vi "JoyStick2.vi"() -> ()   [LabVIEW 2016]
panel:
  in  "JoyStick":bool
  out "X 2":bool
  out "Y 2":bool
  out "Z 2":bool
  out "LowSpeed?":bool
  out "down":string
  out "right":string
  out "Up":string
  out "left":string
  out "Boolean":bool
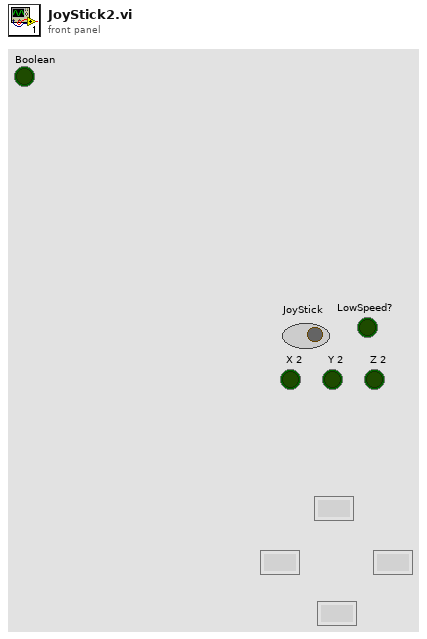
[diagram p1: front panel]
types:
  T1 = typedef "ControllerDiagPacket.ctl" = cluster{"Number of Diag Packets":i32, "Axes":T2[], "error":errorcluster}
  T2 = typedef "AxisDiagPacket.ctl" = cluster{"Axis Name":string, "Analog Input 0":dbl, "Analog Input 1":dbl, "Axis Fault (num)":i32, "Axis Fault (str)":string, "Axis Fault (bits)":cluster{"AmplifierFault":bool, "AmplifierTemperatureFault":bool, "CcwEndOfTravelLimitFault":bool, "CcwSoftwareLimitFault":bool, "CommunicationLostFault":bool, "CwEndOfTravelLimitFault":bool, "CwSoftwareLimitFault":bool, "EmergencyStopFault":bool, "EncoderFault":bool, "ExternalFault":bool, "FeedbackScalingFault":bool, "GantryMisalignFault ":bool, "HallSensorFault":bool, "InPositionTimeoutFault":bool, "InternalFault":bool, "MarkerSearchFault":bool, "MaxVelocityCommandFault":bool, "MissedInterruptFault":bool, "MotorTemperatureFault":bool, "None":bool, "OverCurrentFault":bool, "PositionErrorFault":bool, "PositionFeedbackFault":bool, "PowerSupplyFault":bool, "ProbeInputFault":bool, "SafeZoneFault":bool, "VelocityErrorFault":bool, "VelocityFeedbackFault":bool, "VoltageClampFault":bool}, "Axis Status (num)":i32, "Axis Status (str)":string, "Axis Status (bits)":cluster{"BacklashActive":bool, "CalibrationEnabled1D":bool, "CalibrationEnabled2D":bool, "CommandValid":bool, "DriveAbortPending":bool, "DrivePending":bool, "Enabling":bool, "GainMappingEnabled":bool, "GantryAligned":bool, "GantryRealigning":bool, "Homed":bool, "Homing":bool, "IFOVEnabled":bool, "JogGenerating":bool, "Jogging":bool, "JoystickControl":bool, "MasterSlaveControl":bool, "MotionBlocked":bool, "MotionClamped":bool, "MoveDone":bool, "None":bool, "NotVirtual":bool, "Profiling":bool, "Stability0":bool, "Stability1":bool, "TrajectoryFiltering":bool, "WaitDone":bool}, "Current Command":sgl, "Current Error":sgl, "Current Feedback":sgl, "Digital Inputs":i32, "Digital Outputs":i32, "Drive Status":i32, "Drive Status (str)":string, "Drive Status (bits)":cluster{"AccelerationPhase":bool, "AutofocusActive":bool, "BrakeOutput":bool, "CcwEndOfTravelLimitInput":bool, "CosineEncoderError":bool, "CurrentClamp":bool, "CwEndOfTravelLimitInput":bool, "DecelerationPhase":bool, "DualLoopActive":bool, "EmergencyStopInput":bool, "Enabled":bool, "EncoderClipping":bool, "GalvoCalibrationEnabled":bool, "GalvoPowerCorrection":bool, "HallAInput":bool, "HallBInput":bool, "HallCInput":bool, "HighResolutionMode":bool, "HomeLimitInput":bool, "InPosition":bool, "InPosition2":bool, "MarkerInput":bool, "MarkerLatch":bool, "MoveActive":bool, "NoMotorSupply":bool, "None":bool, "PowerLimiting":bool, "ProgrammingFlash":bool, "ProgrammingMXH":bool, "PSOHaltLatch":bool, "ServoControl":bool, "SineEncoderError":bool}, "Position Feedback Auxiliary":dbl, "Position Command":dbl, "Position Error":dbl, "Position Feedback":dbl, "Program Position Command":dbl, "Program Position Error":dbl, "Program Position Feedback":dbl, "Velocity Command":dbl, "Velocity Error":dbl, "Velocity Feedback":dbl}
  T3 = typedef "TaskStatus.ctl" = cluster{"Task Status0 (num)":i32, "Task Status0 (bits)":cluster{"CallbackHoldActive":bool, "CallbackResponding":bool, "CannedFunctionExecuting":bool, "CornerRounding":bool, "FeedHoldActive":bool, "ImmediateConcurrent":bool, "ImmediateExecuting":bool, "InterruptMotionActive":bool, "JoystickActive":bool, "JoystickLowSpeedActive":bool, "None":bool, "PendingAxesStop":bool, "ProbeCycle":bool, "ProgramAssociated":bool, "ProgramControlRestricted":bool, "ProgramReset":bool, "Retrace":bool, "ReturnMotionExecuting":bool, "SingleStepInto":bool, "SingleStepOver":bool, "SoftHomeActive":bool, "SoftwareESTOPActive":bool, "SpindleActive0":bool, "SpindleActive1":bool, "SpindleActive2":bool, "SpindleActive3":bool}, "Task Status0 (str)":string, "Task Status1 (num)":i32, "Task Status1 (bits)":cluster{"AsyncSMCMotionAbortPending":bool, "CannedFunctionPending":bool, "CutterOffsetsDisabling":bool, "CutterOffsetsEnablingNegative":bool, "CutterOffsetsEnablingPositive":bool, "CutterRadiusDisabling":bool, "CutterRadiusEnabling":bool, "FeedHeldAxesStopped":bool, "GalvoIFVDeactivationPending":bool, "IFOVBufferHold":bool, "Interrupted":bool, "MotionModeAbsOffsets":bool, "MSOChange":bool, "NoMFOFloor":bool, "None":bool, "OnGosubPending":bool, "ProgramStopPending":bool, "RetraceRequested":bool, "SpindleFeedHeld":bool}, "Task Status1 (str)":string, "Task Status2 (num)":i32, "Task Status2 (bits)":cluster{"Coord1Plane1":bool, "Coord1Plane2":bool, "Coord1Plane3":bool, "Coord2Plane1":bool, "Coord2Plane2":bool, "Coord2Plane3":bool, "CutterOffsetsActiveNeg":bool, "CutterOffsetsActivePos":bool, "CutterRadiusActiveLeft":bool, "CutterRadiusActiveRight":bool, "LimitFeedRateActive":bool, "LimitMFOActive":bool, "MirrorActive":bool, "MotionContinuousActive":bool, "MotionFiber":bool, "MotionModeCCW":bool, "MotionModeCoordinated":bool, "MotionModeCW":bool, "MotionModeRapid":bool, "MotionPVT":bool, "None":bool, "NormalcyActiveLeft":bool, "NormalcyActiveRight":bool, "NormalcyAlignment":bool, "OffsetFixtureActive":bool, "ProfileActive":bool, "RotationActive":bool, "RThetaCylindricalActive":bool, "RThetaPolarActive":bool, "ScalingActive":bool}, "Task Status2 (str)":string, "Task Mode (num)":i32, "Task Mode (bits)":cluster{"Absolute":bool, "AccelModeRate":bool, "AccelTypeLinear":bool, "AccelTypeScurve":bool, "AutoMode":bool, "BlockDelete":bool, "BlockDelete2":bool, "DecelModeRate":bool, "DecelTypeLinear":bool, "DecelTypeScurve":bool, "InverseCircular":bool, "InverseDominance":bool, "MFOActiveOnJog":bool, "MFOLock":bool, "Minutes":bool, "MotionContinuous":bool, "MSOLock":bool, "None":bool, "OptionalPause":bool, "OverMode":bool, "ProgramFeedRateMPU":bool, "ProgramFeedRateUPR":bool, "Secondary":bool, "SpindleStopOnProgramHalt":bool, "WaitAuto":bool, "WaitForInPos":bool}, "Task Mode (str)":string, "Queue Status (num)":i32, "Queue Status (bits)":cluster{"None":bool, "QueueBufferEmpty":bool, "QueueBufferFull":bool, "QueueBufferPaused":bool, "QueueBufferStarted":bool, "QueueLargeProgramExecuting":bool, "QueueModeActive":bool}, "Queue Status (str)":string, "Task State":i32}
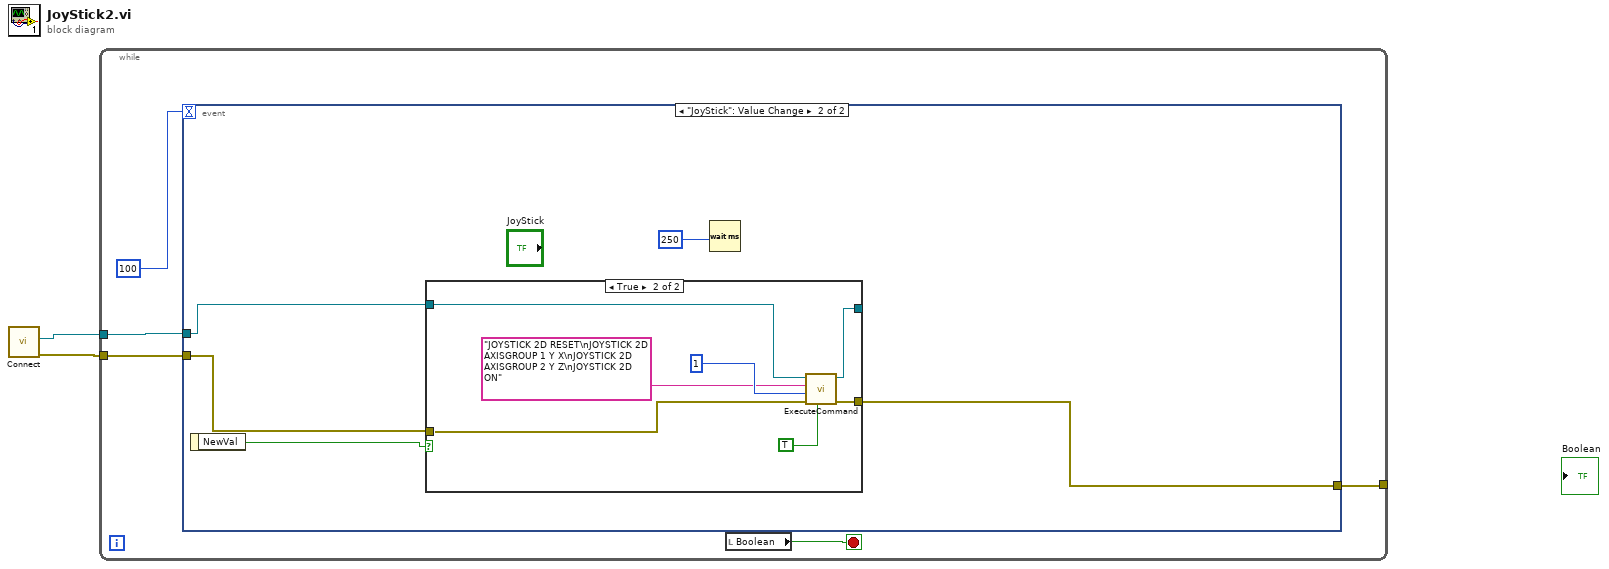
[diagram p0: block diagram]
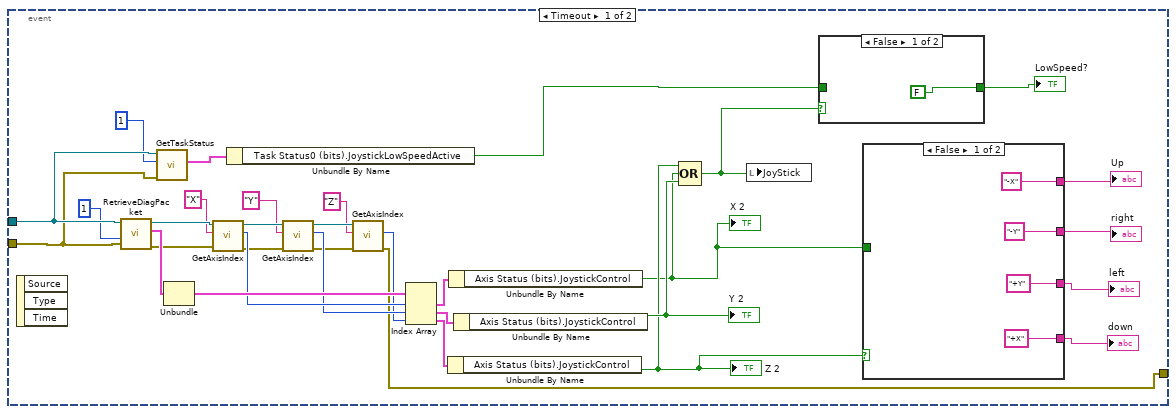
[diagram p2: hidden frame]
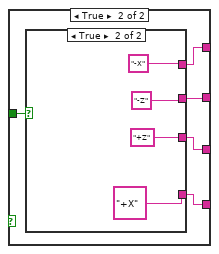
[diagram p4: hidden frame]
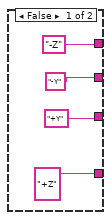
[diagram p5: hidden frame]
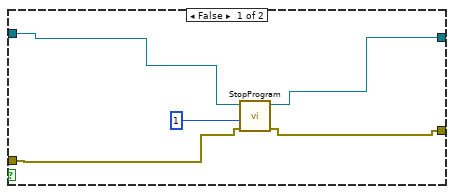
[diagram p6: hidden frame]
diagram:
  n1 = call "Connect.vi"() -> ("error out"=w1:errorcluster, "controller"=w2:refnum<k24>)  [unwired: 10 in]
  n2 = while {
    tunnel: w2 -> [w7]
    tunnel: w1 -> [w4]
    tunnel: [w3] -> _
    stop <- w6 stop-if-true
    n3 = event shown="[1] \"JoyStick\": Value Change" {
      selector: _ -> [_ _]
      dyn-events: _ -> [_ _]
      timeout: 100 -> [_ _]
      tunnel: w7 -> [w29 w61]
      tunnel: w4 -> [w12 w63]
      tunnel: [w8 w60] -> w3
      event Timeout {
        n4 = event-data() -> ()  [unwired: 1 in, 3 out]
        n5 = call "RetrieveDiagPacket.vi"("error in (no error)"=w12, "axisMask"=1, "Controller In"=w29) -> ("error out"=w15:errorcluster, "ControllerDiagPacket"=w36:T1, "Controller Out"=w40:refnum<k24>)  [unwired: 6 in]
        n6 = call "GetTaskStatus.vi"("error in (no error)"=w12, "task"=1, "controller in"=w29) -> ("task status"=w28:T3)  [unwired: 6 in, 2 out]
        n7 = Unbundle(w36) -> ("Axes"=w35:T2[])  [unwired: 2 out]
        n8 = call "GetAxisIndex.vi"("error in (no error)"=w15, "axis name"="X", "controller in"=w40) -> ("error out"=w14:errorcluster, "axis index"=w34:i32, "controller out"=w39:refnum<k24>)  [unwired: 6 in]
        n9 = Unbundle By Name(w28) -> ("Task Status0 (bits).JoystickLowSpeedActive"=w11:bool)
        n10 = call "GetAxisIndex.vi"("error in (no error)"=w14, "axis name"="Y", "controller in"=w39) -> ("error out"=w13:errorcluster, "axis index"=w33:i32, "controller out"=w37:refnum<k24>)  [unwired: 6 in]
        n11 = call "GetAxisIndex.vi"("error in (no error)"=w13, "axis name"="Z", "controller in"=w37) -> ("error out"=w8:errorcluster, "axis index"=w23:i32)  [unwired: 6 in, 1 out]
        n12 = Index Array(array=w35, index #1=w34, index #2=w33, index #3=w23) -> (element #1=w32:T2, element #2=w31:T2, element #3=w30:T2)
        n13 = Unbundle By Name(w30) -> ("Axis Status (bits).JoystickControl"=w21:bool)
        "Z 2" <- w21
        n14 = Unbundle By Name(w32) -> ("Axis Status (bits).JoystickControl"=w16:bool)
        "X 2" <- w16
        n15 = Unbundle By Name(w31) -> ("Axis Status (bits).JoystickControl"=w22:bool)
        "Y 2" <- w22
        n16 = Compound Arithmetic op=OR(w21, w16, w22) -> (w9:bool)
        n17 = local write "JoyStick"(w9) -> ()
        n18 = case shown="False" w9 {
          tunnel: w11 -> [_ w42]
          tunnel: [FALSE w42] -> w10
          frame False {
          }
          frame True {
          }
        }
        "LowSpeed?" <- w10
        n19 = case shown="False" w21 {
          tunnel: ["-X" w47] -> w20
          tunnel: ["-Y" w48] -> w19
          tunnel: ["+Y" w49] -> w18
          tunnel: ["+X" w50] -> w17
          tunnel: w16 -> [_ w51]
          frame False {
          }
          frame True {
            n20 = case shown="True" w51 {
              tunnel: ["-Z" "-X"] -> w47
              tunnel: ["-Y" "-Z"] -> w48
              tunnel: ["+Y" "+Z"] -> w49
              tunnel: ["+Z" "+X"] -> w50
              frame False {
              }
              frame True {
              }
            }
          }
        }
        "down" <- w17
        "right" <- w19
        "Up" <- w20
        "left" <- w18
      }
      event "JoyStick": Value Change {
        n21 = event-data() -> ("NewVal"=w62:bool)  [unwired: 1 in]
        n22 = case shown="True" w62 {
          tunnel: w61 -> [w69 w75]
          tunnel: w63 -> [w67 w72]
          tunnel: [w66 w71] -> w60
          tunnel: [w65 w70] -> _
          frame False {
            n23 = call "StopProgram.vi"("error in (no error)"=w67, "taskId"=1, "controller in"=w69) -> ("error out"=w66:errorcluster, "controller out"=w65:refnum<k24>)  [unwired: 7 in]
          }
          frame True {
            n24 = call "ExecuteCommand.vi"("return immediately"=TRUE, "error in (no error)"=w72, "taskId"=1, "Command Code"="JOYSTICK 2D RESET\nJOYSTICK 2D AXISGROUP 1 Y X\nJOYSTICK 2D AXISGROUP 2 Y Z\nJOYSTICK 2D ON", "controller in"=w75) -> ("error out"=w71:errorcluster, "controller out"=w70:refnum<k24>)  [unwired: 4 in, 1 out]
          }
        }
        n25 = Wait (ms)(milliseconds to wait=250) -> ()  [unwired: 1 out]
      }
    }
    n26 = local read "Boolean"() -> (w6:bool)
  }
